vi "TouchEvent.vi"(9 "IA State":T1) -> (1 "id":dbl, 2 "Toque":bool)   [LabVIEW 2016]
uses:
  Core/AI Input.ctl
  Core/AI Robot.ctl
  Intel/Functions Enum.ctl
  Core/AI Ball.ctl
  Core/Field Size.ctl
  Core/AI Judge.ctl
  Intel/Command Enum.ctl
panel:
  in  "Dist Para Toque":dbl=110.0
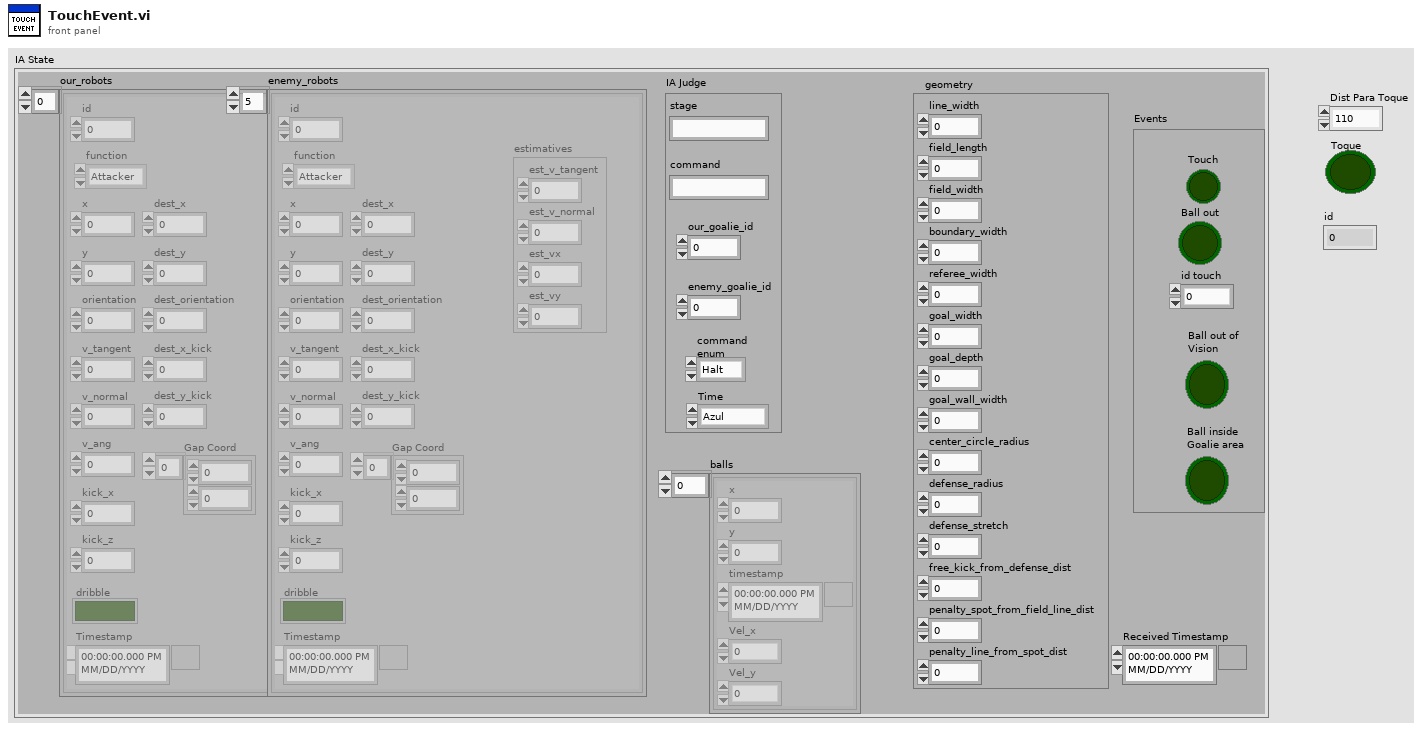
[diagram p1: front panel]
types:
  T1 = typedef "AI Input.ctl" = cluster{"our_robots":T2[], "enemy_robots":T2[], "balls":T4[], "geometry":T5, "IA Judge":T6, "Received Timestamp":timestamp, "Events":cluster{"Touch":bool, "Ball out":bool, "id touch":dbl, "Ball out of \nVision":bool, "Ball inside \nGoalie area":bool}}
  T2 = typedef "AI Robot.ctl" = cluster{"id":u32, "function":T3, "x":dbl, "y":dbl, "orientation":dbl, "v_tangent":dbl, "v_normal":dbl, "v_ang":dbl, "kick_x":dbl, "kick_z":dbl, "dribble":bool, "Timestamp":timestamp, "dest_x":dbl, "dest_y":dbl, "dest_orientation":dbl, "estimatives":cluster{"est_v_tangent":dbl, "est_v_normal":dbl, "est_vx":dbl, "est_vy":dbl}, "dest_x_kick":dbl, "dest_y_kick":dbl, "Gap Coord":dbl[]}
  T3 = typedef "Functions Enum.ctl" = enum16{"Attacker", "Goalie", "Defender", "Striker", "Goto 0", "Dummy", "ZigZag"}
  T4 = typedef "AI Ball.ctl" = cluster{"x":dbl, "y":dbl, "timestamp":timestamp, "Vel_x":dbl, "Vel_y":dbl}
  T5 = typedef "Field Size.ctl" = cluster{"line_width":u32, "field_length":u32, "field_width":u32, "boundary_width":u32, "referee_width":u32, "goal_width":u32, "goal_depth":u32, "goal_wall_width":u32, "center_circle_radius":u32, "defense_radius":u32, "defense_stretch":u32, "free_kick_from_defense_dist":u32, "penalty_spot_from_field_line_dist":u32, "penalty_line_from_spot_dist":u32}
  T6 = typedef "AI Judge.ctl" = cluster{"stage":string, "command":string, "our_goalie_id":dbl, "enemy_goalie_id":dbl, "command\nenum":T7, "Time":enum16{"Azul", "Amarelo"}}
  T7 = typedef "Command Enum.ctl" = enum16{"Halt", "Stop", "Force Start", "PKA Normal Start", "Prepare Kickoff Ally", "PKE Normal Start", "Prepare Kickoff Enemy", "Prepare Penalty Ally", "PPA Normal Start", "Prepare Penalty Enemy", "PPE Normal Start", "Direct Free Enemy", "Direct Free Ally", "Indirect Free Enemy", "Indirect Free Ally", "Timeout Enemy", "Timeout Ally", "Goal Enemy", "Goal Ally", "Ball Placement Enemy", "Ball Placement Ally", "None"}
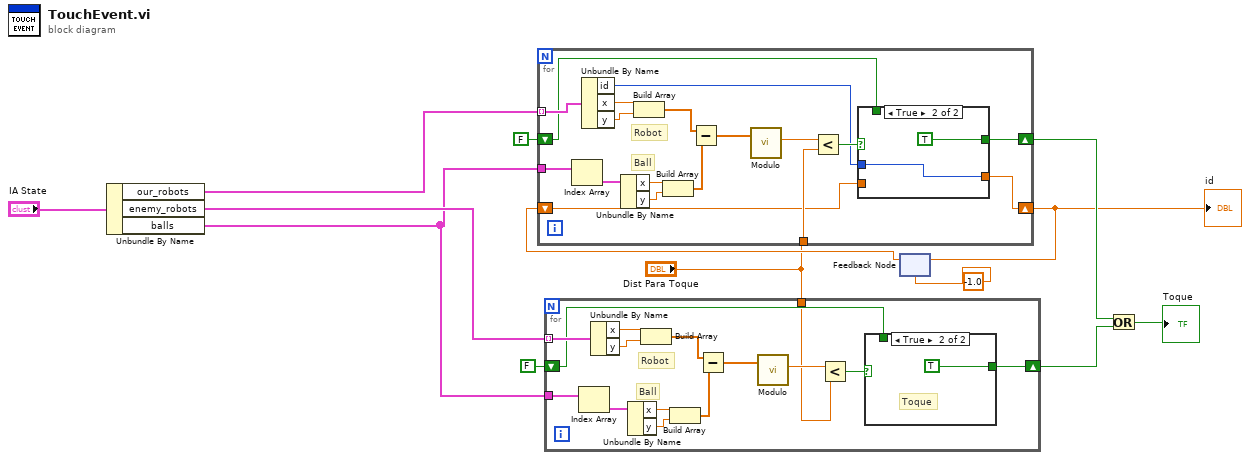
[diagram p0: block diagram]
diagram:
  n1 = Unbundle By Name("IA State") -> ("our_robots"=w5:T2[], "enemy_robots"=w9:T2[], "balls"=w8:T4[])
  n2 = for {
    tunnel: w9 -> [w24] mode=indexing
    tunnel: w8 -> [w28]
    shift-right: [w16] -> w7
    shift-left: FALSE -> [w15]
    tunnel: "Dist Para Toque" -> [w14]
    # "Ball"
    # "Robot"
    n3 = Index Array(array=w28) -> (element=w27:T4)  [unwired: 1 in]
    n4 = Unbundle By Name(w24) -> ("x"=w23:dbl, "y"=w22:dbl)
    n5 = Unbundle By Name(w27) -> ("x"=w26:dbl, "y"=w25:dbl)
    n6 = Build Array(w23, w22) -> (w21:dbl[])
    n7 = Build Array(w26, w25) -> (w20:dbl[])
    n8 = Subtract(x=w21, y=w20) -> (x-y=w19:dbl[])
    n9 = call "Modulo.vi"("2D vector"=w19) -> ("Modulo"=w17:dbl)  [unwired: 10 in]
    n10 = Less?(x=w17, y=w14) -> (x < y?=w18:bool)
    n11 = case shown="True" w18 {
      tunnel: [w29 TRUE] -> w16
      tunnel: w15 -> [w29 _]
      frame False {
        # "Sem toque"
      }
      frame True {
        # "Toque"
      }
    }
  }
  n12 = feedback #1(-1.0) -> (w3:dbl)
  n13 = for {
    tunnel: w5 -> [w44] mode=indexing
    tunnel: w8 -> [w48]
    shift-right: [w36] -> w11
    shift-left: FALSE -> [w35]
    tunnel: "Dist Para Toque" -> [w34]
    shift-right: [w33] -> w4
    shift-left: w3 -> [w31]
    # "Ball"
    # "Robot"
    n14 = Index Array(array=w48) -> (element=w47:T4)  [unwired: 1 in]
    n15 = Unbundle By Name(w44) -> ("id"=w32:u32, "x"=w43:dbl, "y"=w42:dbl)
    n16 = Unbundle By Name(w47) -> ("x"=w46:dbl, "y"=w45:dbl)
    n17 = Build Array(w43, w42) -> (w41:dbl[])
    n18 = Build Array(w46, w45) -> (w40:dbl[])
    n19 = Subtract(x=w41, y=w40) -> (x-y=w39:dbl[])
    n20 = call "Modulo.vi"("2D vector"=w39) -> ("Modulo"=w37:dbl)  [unwired: 10 in]
    n21 = Less?(x=w37, y=w34) -> (x < y?=w38:bool)
    n22 = case shown="True" w38 {
      tunnel: [w50 TRUE] -> w36
      tunnel: w35 -> [w50 _]
      tunnel: [w49 w51] -> w33
      tunnel: w32 -> [_ w51]
      tunnel: w31 -> [w49 _]
      frame False {
      }
      frame True {
      }
    }
  }
  "id" <- w4
  n23 = feedback-in #1(w4) -> ()
  n24 = Or(x=w11, y=w7) -> (x .or. y?=→"Toque":bool)
